vi "DatabaseHand_FindSubGroup.vi"(8 "error in (no error)":errorcluster, 10 "group":string, 11 "Database RefNum in":T2) -> (0 "error out":errorcluster, 1 "group found":T1[](array[typedef]), 3 "Database RefNum out":T2)   [LabVIEW 2016]
doc: "This VI finds the RefNum of an existing object with the input Name or creates a new object if the Name is not found or Name is unwired or an empty string.\nCopyright 2001 VI Engineering, Inc."
uses:
  DatabaseHand_RefNum.ctl
  DatabaseHan_DatabaseElement.ctl
  DatabaseHand_Function.ctl
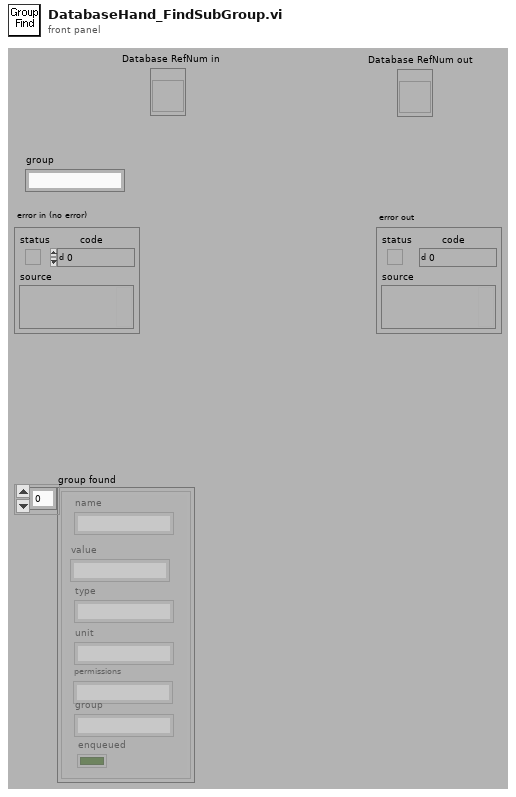
[diagram p1: front panel]
types:
  T1 = typedef "DatabaseHan_DatabaseElement.ctl" = cluster{"name":string, "value":string, "type":string, "unit":string, "permissions":string, "enqueued":bool, "group":string}
  T2 = typedef "DatabaseHand_RefNum.ctl" = refnum<vi>
  T3 = typedef "DatabaseHand_Function.ctl" = enum16{"Reset", "Register", "Get Data", "Set Data", "Unregister", "Test", "Get Objects", "Delete Data"}
  T4 = typedef "Database_Refnum.ctl" = refnum<vi>
  T5 = typedef "DatabaseHand_Element.ctl" = cluster{"name":string, "Database":T1[]}
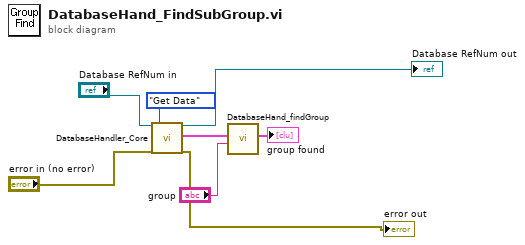
[diagram p0: block diagram]
diagram:
  n1 = call "DatabaseHandler_Core.vi"("Object Refnum In"="Database RefNum in", "error in (no error)"="error in (no error)", "Function (Get Data)"=DatabaseHand_Function."Get Data") -> ("Object Refnum out"=→"Database RefNum out":T4, "Object Data Out"=w1:T5, "error out"=→"error out":errorcluster)  [unwired: 4 in, 10 out]
  n2 = call "DatabaseHand_findGroup.vi"("group"="group", "Data In"=w1) -> ("group"=→"group found":T1[])  [unwired: 9 out]
